vi "Laba1.vi"() -> ()   [LabVIEW 2018]
panel:
  out "Numeric":dbl
  out "XY Graph":cluster{"X":dbl, "Y":dbl}[](graph)
  out "S":dbl
  in  "node c":dbl
  in  "node b":dbl
  in  "node a":dbl
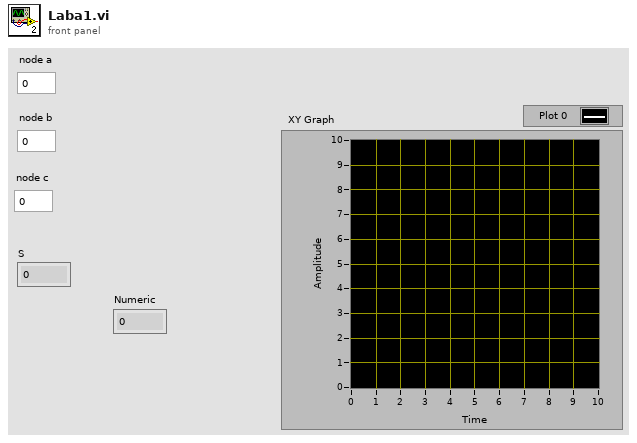
[diagram p1: front panel]
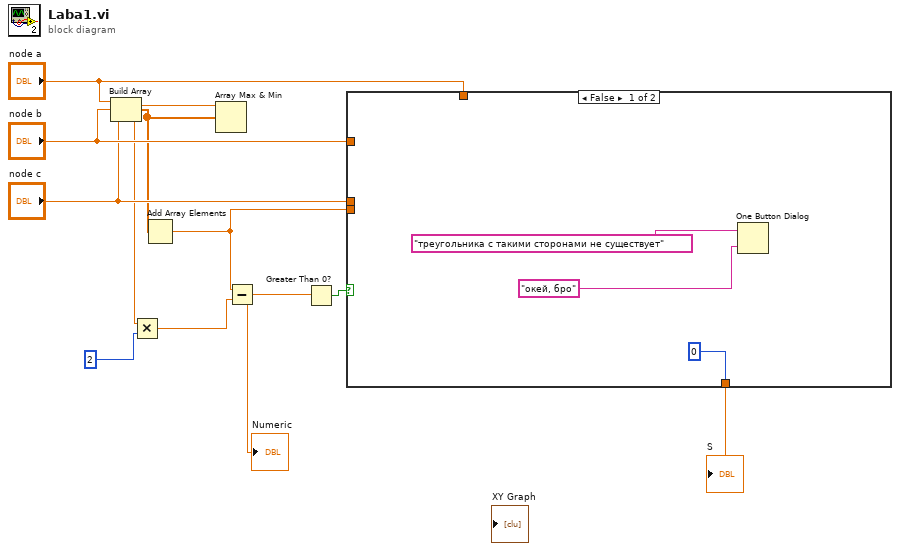
[diagram p0: block diagram]
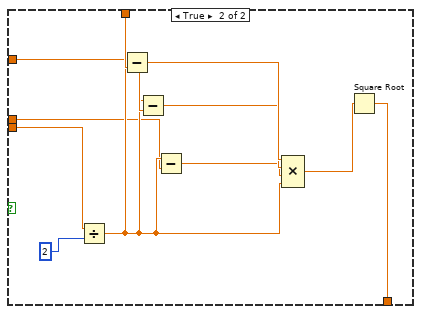
[diagram p2: hidden frame]
diagram:
  n1 = Build Array("node a", "node b", "node c") -> (w7:dbl[])
  n2 = Add Array Elements(numeric array=w7) -> (sum=w11:dbl)
  n3 = Array Max & Min(array=w7) -> (max value=w2:dbl)  [unwired: 3 out]
  n4 = Multiply(x=w2, y=2) -> (x*y=w1:dbl)
  n5 = Subtract(x=w11, y=w1) -> (x-y=w5:dbl)
  "Numeric" <- w5
  n6 = Greater Than 0?(x=w5) -> (x > 0?=w4:bool)
  n7 = case shown="False" w4 {
    tunnel: w11 -> [_ w24]
    tunnel: "node a" -> [_ w23]
    tunnel: "node b" -> [_ w21]
    tunnel: "node c" -> [_ w18]
    tunnel: [0 w15] -> w6
    frame False {
      n8 = One Button Dialog(message="треугольника с такими сторонами не существует", button name ("OK")="окей, бро") -> ()  [unwired: 1 out]
    }
    frame True {
      n9 = Divide(x=w24, y=2) -> (x/y=w19:dbl)
      n10 = Subtract(x=w19, y=w23) -> (x-y=w22:dbl)
      n11 = Subtract(x=w19, y=w21) -> (x-y=w20:dbl)
      n12 = Subtract(x=w19, y=w18) -> (x-y=w17:dbl)
      n13 = Compound Arithmetic op=MULTIPLY(w22, w20, w17, w19) -> (w16:dbl)
      n14 = Square Root(x=w16) -> (sqrt(x)=w15:dbl)
    }
  }
  "S" <- w6
